vi "_queueName.vi"() -> ()   [LabVIEW 2020, in "main.lvlib"]
uses:
  main.lvlib
panel:
  in  "main":string="main"
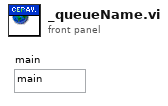
[diagram p1: front panel]
diagram:
